vi "Animation.vi"() -> ()   [LabVIEW 2015]
panel:
  in  "Break":bool
  in  "Play":bool
  in  "Frames Per Second":u32(slide)=30 scale=1.0..60.0
  out "Picture Ring":u16(ring)
  in  "stop":bool
  # "Virtual Instrumentation Lab - Spring 2015 - Final Project - Abhishek Barla"
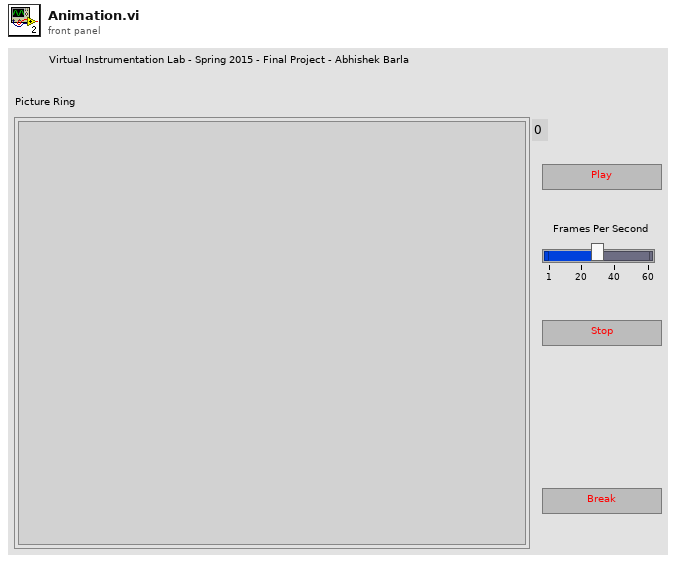
[diagram p1: front panel]
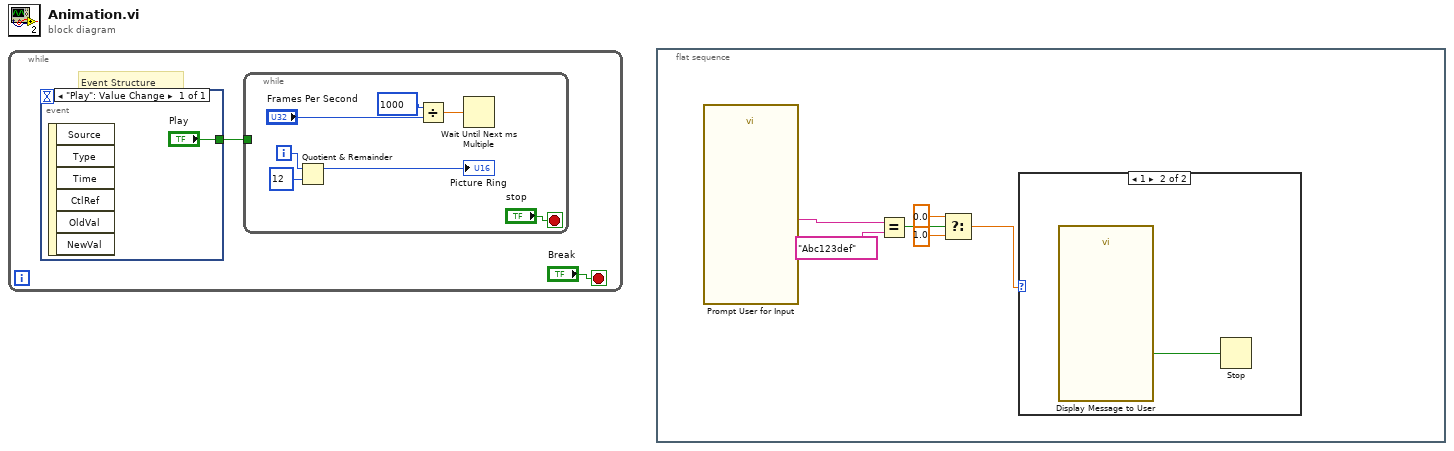
[diagram p0: block diagram]
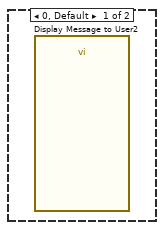
[diagram p2: hidden frame]
diagram:
  n1 = while {
    stop <- "Break" stop-if-true
    # "Event Structure"
    n2 = event shown="[0] \"Play\": Value Change" {
      selector: _ -> [_]
      dyn-events: _ -> [_]
      timeout: _ -> [_]
      tunnel: ["Play"] -> w2
      event "Play": Value Change {
        n3 = event-data() -> ()  [unwired: 1 in, 6 out]
      }
    }
    n4 = while {
      tunnel: w2 -> [_]
      i -> [w4]
      stop <- "stop" stop-if-true
      n5 = Quotient & Remainder(x=w4, y=12) -> (x-y*floor(x/y)=→"Picture Ring":i32)  [unwired: 1 out]
      n6 = Divide(x=u32 1000, y="Frames Per Second") -> (x/y=w6:dbl)
      n7 = Wait Until Next ms Multiple(millisecond multiple=w6) -> ()  [unwired: 1 out]
    }
  }
  n8 = flat-sequence {
    frame #0 {
      n9 = call "Prompt User for Input"() -> ("Enter Here:"=w16:string)  [unwired: 17 in, 2 out]
      n10 = Equal?(x=w16, y="Abc123def") -> (x = y?=w14:bool)
      n11 = Select(t=0.0, s=w14, f=1.0) -> (s? t:f=w13:dbl)
      n12 = case shown="1" w13 {
        frame 0, Default {
          n13 = call "Display Message to User2"() -> ()  [unwired: 10 in, 2 out]
        }
        frame 1 {
          n14 = call "Display Message to User"() -> ("OK"=w17:bool)  [unwired: 10 in, 1 out]
          n15 = Stop(stop? (T)=w17) -> ()
        }
      }
    }
  }
